vi "DELETE_LOG_FILE.vi"(8 "error in (no error)":errorcluster, 11 "Log File Name":string) -> (0 "error out":errorcluster)   [LabVIEW 2019]
uses:
  Typedefs/Message.ctl
  Typedefs/Sensor Types.ctl
  Typedefs/Message Types.ctl
  Message Globals.vi
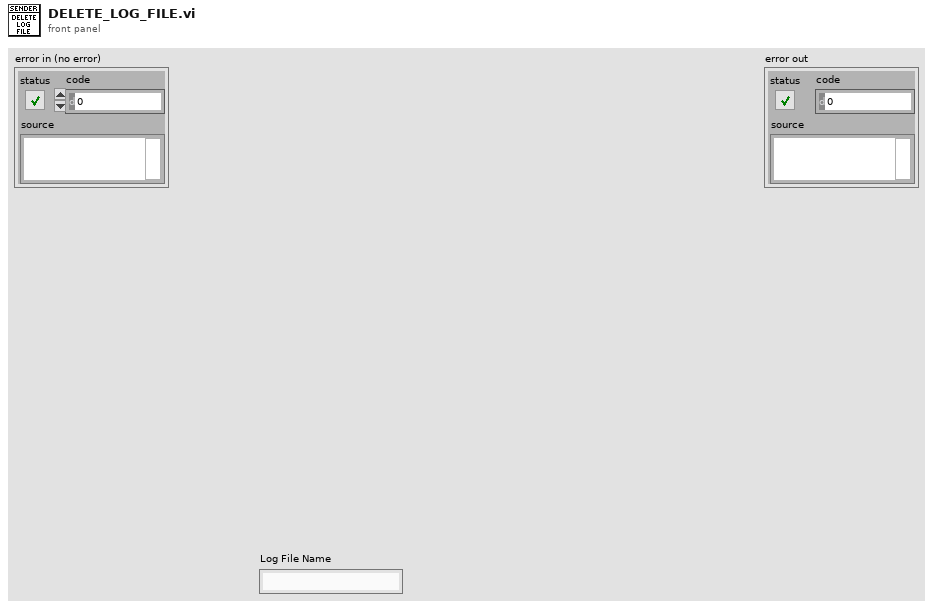
[diagram p1: front panel]
types:
  T1 = typedef "Message Types.ctl" = enum16{"HEART_BEAT", "CONNECT", "GET_CURRENT_MEASUREMENTS", "GET_LOG_FILE", "SEND_LOG_FILE_SIZE", "SEND_LOG_FILE_CHUNK", "GET_LOGGING_PERIOD", "SET_LOGGING_PERIOD", "SEND_SD_CARD_INFO", "GET_LOGS_LIST", "SEND_LOG_FILE_NAME", "SEND_LOGGING_PERIOD", "GET_RTC_TIME", "SET_RTC_TIME", "SEND_RTC_TIME", "SEND_CURRENT_MEASUREMENTS", "DELETE_LOG_FILE", "GET_SD_CARD_INFO", "GET_BATTERY_INFO", "SEND_BATTERY_INFO", "GET_LOG_FILE_SIZE", "ERROR_MSG"}
  T2 = typedef "Message.ctl" = cluster{"Payload Size":u8, "Sequence Number":u8, "Sensor Type":T3, "Message Types":T1, "Data":u8[]}
  T3 = typedef "Sensor Types.ctl" = enum16{"APP", "TURBIDITY", "PH"}
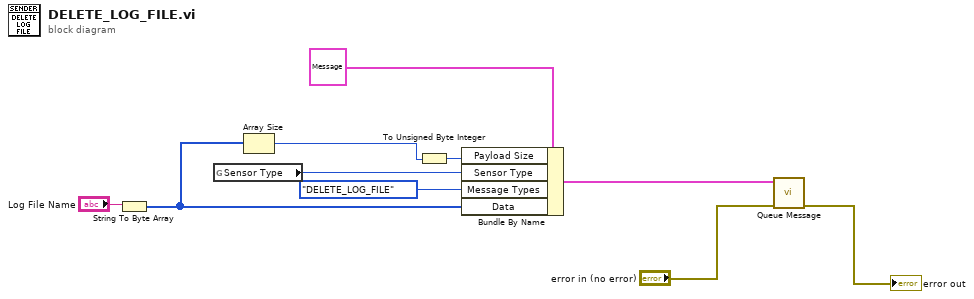
[diagram p0: block diagram]
diagram:
  n1 = String To Byte Array(string="Log File Name") -> (unsigned byte array=w6:u8[])
  n2 = global read "Message Globals.vi" "Sensor Type"() -> (w7:T3)
  n3 = Array Size(array=w6) -> (size(s)=w4:i32)
  n4 = To Unsigned Byte Integer(number=w4) -> (unsigned 8bit integer=w5:u8)
  n5 = Bundle By Name(cluster=T2 {"Payload Size"=0, "Sequence Number"=0, "Sensor Type"=enum."APP", "Message Types"=enum."HEART_BEAT", "Data"=[]} ("Message"), "Payload Size"=w5, "Sensor Type"=w7, "Message Types"=Message_Types."DELETE_LOG_FILE", "Data"=w6) -> (w3:T2)
  n6 = call "Queue Message.vi"("error in (no error)"="error in (no error)", "Message"=w3) -> ("error out"=→"error out":errorcluster)  [unwired: 9 in]
